vi "Add.vi"(8 "error in (no error)":errorcluster, 10 "Child in":refnum<class "3D Object.lvclass">, 11 "Parent in":refnum<class "3D Object.lvclass">) -> (0 "error out":errorcluster, 2 "Child out":refnum<class "3D Object.lvclass">, 3 "Parent out":refnum<class "3D Object.lvclass">)   [LabVIEW 2015, in "3D Object.lvclass"]
uses:
  3D Object.lvclass
  3D Object.lvclass/3D Object.ctl
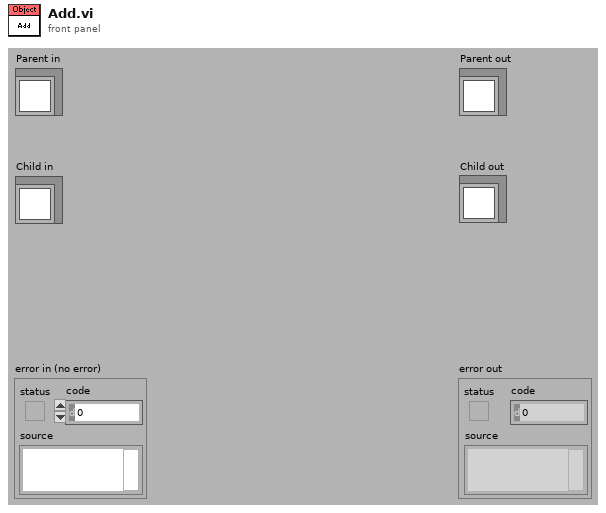
[diagram p1: front panel]
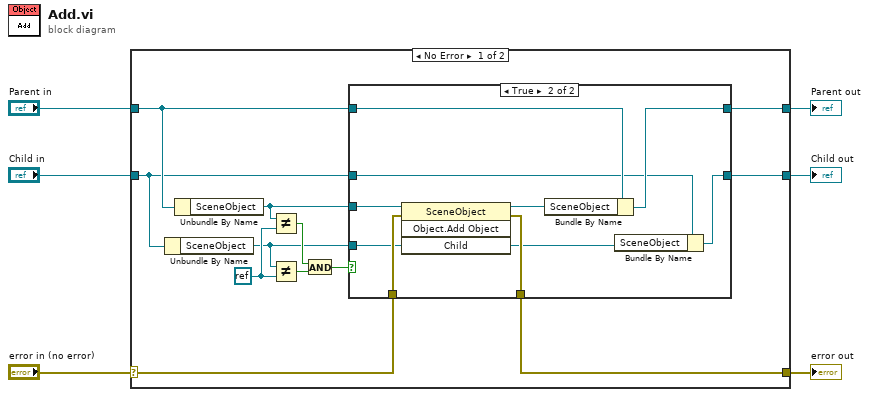
[diagram p0: block diagram]
diagram:
  n1 = case shown="No Error" "error in (no error)" {
    selector: "error in (no error)" -> [w18 w34]
    tunnel: [w17 w34] -> w5
    tunnel: [w15 w33] -> w3
    tunnel: "Parent in" -> [w16 w33]
    tunnel: "Child in" -> [w14 w32]
    tunnel: [w13 w32] -> w1
    frame No Error {
      w11 = refnum<k0> refnum
      n2 = Unbundle By Name(w14) -> ("SceneObject"=w8:refnum<vi>)
      n3 = Unbundle By Name(w16) -> ("SceneObject"=w12:refnum<vi>)
      n4 = Not Equal?(x=w12, y=w11) -> (x != y?=w9:bool)
      n5 = Not Equal?(x=w8, y=w11) -> (x != y?=w10:bool)
      n6 = And(x=w9, y=w10) -> (x .and. y?=w7:bool)
      n7 = case shown="True" w7 {
        tunnel: w18 -> [w19 w31]
        tunnel: [w19 w30] -> w17
        tunnel: w16 -> [w21 w27]
        tunnel: [w21 w26] -> w15
        tunnel: w14 -> [w20 w25]
        tunnel: [w20 w24] -> w13
        tunnel: w12 -> [_ w23]
        tunnel: w8 -> [_ w22]
        frame False {
        }
        frame True {
          n8 = invoke class="SceneObject" method="Object.Add Object"(reference=w23, error in=w31, "Child"=w22) -> (reference out=w28:refnum<vi>, error out=w30:errorcluster, "Child"=w29:refnum<vi>)  [unwired: 1 in, 1 out]
          n9 = Bundle By Name(cluster=w27, "SceneObject"=w28) -> (w26:refnum<class "3D Object.lvclass">)
          n10 = Bundle By Name(cluster=w25, "SceneObject"=w29) -> (w24:refnum<class "3D Object.lvclass">)
        }
      }
    }
    frame Error {
    }
  }
  "error out" <- w5
  "Parent out" <- w3
  "Child out" <- w1
